vi "List Buckets.vi"() -> ()   [LabVIEW 2015]
doc: "Demonstrates how to list all of the Amazon S3 buckets you own."
uses:
  Core/HTTP Request/AWS Credentials.ctl
  Bucket/Bucket.lvclass/Bucket.ctl
  Bucket/Read Name.vi
  Bucket/Read Creation Date.vi
  Bucket/Bucket.lvclass
  Core/HTTP Request/HTTP Request.lvclass
panel:
  in  "Secret Key":string
  in  "Access Key":string
  out "Buckets":i32(listbox)
  # "Overview: Demonstrates how to list all Amazon S3 buckets created by an authenticated user.\nRequirements: LabVIEW AWS Toolkit and a registered Amazon AWS account\nInstructions:\n1. Specify the Access Key and Secret Key for your AWS account. You can create an account at http://aws.amazon.com.\n2. Run the VI. All the buckets associated with your account should be listed in the Buckets indicator."
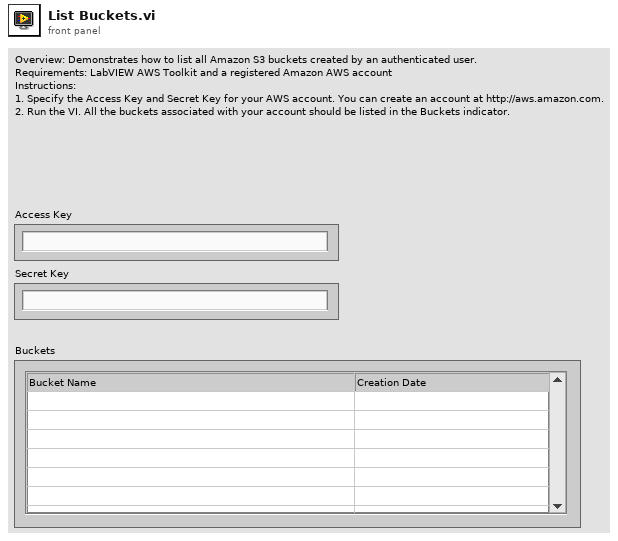
[diagram p1: front panel]
types:
  T1 = typedef "NI_AWS_Core.lvlib/HTTP Request.lvclass/AWS Credentials.ctl" = cluster{"Access Key":string, "Secret Key":string}
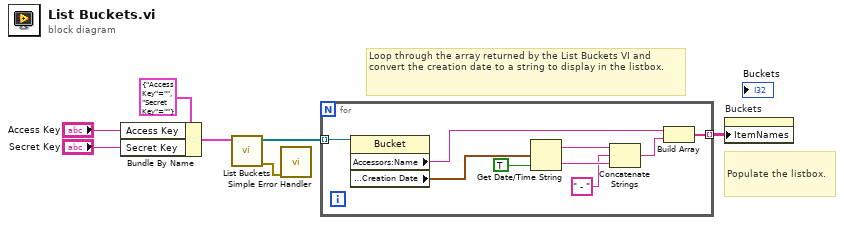
[diagram p0: block diagram]
diagram:
  # "Populate the listbox."
  # "Loop through the array returned by the List Buckets VI and convert the creation date to a string to display in the listbox."
  n1 = Bundle By Name(cluster=T1 {"Access Key"="", "Secret Key"=""} ("AWS Credentials in"), "Access Key"="Access Key", "Secret Key"="Secret Key") -> (w1:T1)
  n2 = call "List Buckets.vi"("AWS Credentials"=w1) -> ("error out"=w2:errorcluster, "Buckets"=w7:refnum<class "Bucket.lvclass">[])  [unwired: 7 in, 2 out]
  n3 = call <vilib>:"Simple Error Handler.vi"("error in (no error)"=w2) -> ()  [unwired: 4 in, 5 out]
  n4 = for {
    tunnel: w7 -> [w16] mode=indexing
    tunnel: [w10] -> w6 mode=indexing
    n5 = property class="Bucket"(reference=w16) -> ("Accessors:Name"=w8:string, "Accessors:Creation Date"=w9:timestamp)  [unwired: 1 in, 2 out]
    n6 = Get Date/Time String(seconds (now)=w9, want seconds? (F)=TRUE) -> (date string=w14:string, time string=w13:string)  [unwired: 1 in]
    n7 = Concatenate Strings(w14, " - " ("string"), w13) -> (w11:string)
    n8 = Build Array(w8, w11) -> (w10:string[])
  }
  n9 = property on="Buckets" class="MCListbox (strict)"("ItemNames"=w6) -> ()  [unwired: 2 in, 2 out]
